vi "OnImageFrameAvailable Event Callback - TLCamera Main Color.vi"(4 "User Parameter":T3, 5 "Event Data":T4, 6 "Control Ref":refnum<k24>, 7 "Event Common Data":T5) -> ()   [LabVIEW 2015]
uses:
  C:/code/Host/Installer/Scientific Camera Interfaces/LabVIEW/32_bit/Library_X86/Thorlabs.TSI.TLCameraInterfaces.dll
  32_bit/Library_X86/Thorlabs.TSI.TLCameraInterfaces.dll
  SubVIs/Parameters Get & Set/Get Parameters/Get ColorFilterArrayPhase.vi
  C:/code/Host/Installer/Scientific Camera Interfaces/LabVIEW/32_bit/Library_X86/Thorlabs.TSI.ImageDataInterfaces.dll
  32_bit/Library_X86/Thorlabs.TSI.ImageDataInterfaces.dll
  SubVIs/Parameters Get & Set/Get Parameters/Get CameraSensorType.vi
  Controls/Color Modes.ctl
  C:/code/Host/Installer/Scientific Camera Interfaces/LabVIEW/32_bit/Library_X86/Thorlabs.TSI.Demosaicker.dll
  32_bit/Library_X86/Thorlabs.TSI.Demosaicker.dll
  C:/code/Host/Installer/Scientific Camera Interfaces/LabVIEW/32_bit/Library_X86/Thorlabs.TSI.ColorProcessor.dll
  32_bit/Library_X86/Thorlabs.TSI.ColorProcessor.dll
  C:/code/Host/Installer/Scientific Camera Interfaces/LabVIEW/32_bit/Library_X86/Thorlabs.TSI.ColorInterfaces.dll
  32_bit/Library_X86/Thorlabs.TSI.ColorInterfaces.dll
  SubVIs/Color/Color Processor References.ctl
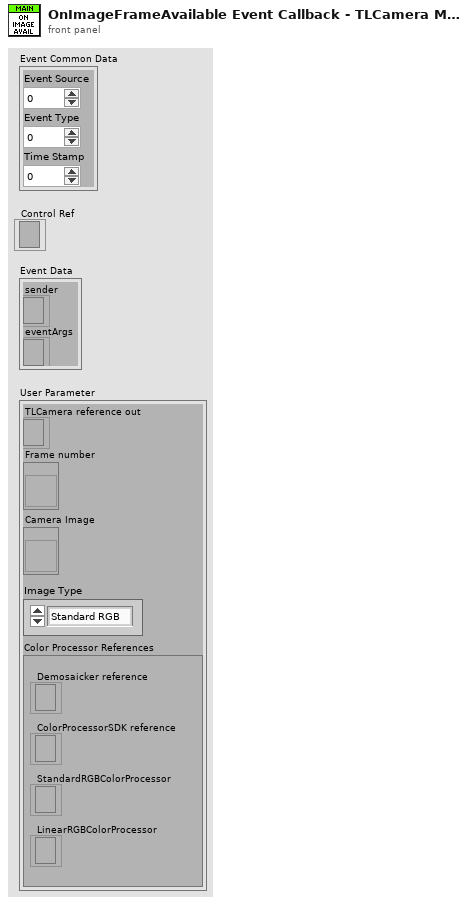
[diagram p1: front panel]
types:
  T1 = typedef "Color Modes.ctl" = enum16{"Standard RGB", "Linear RGB", "Unprocessed"}
  T2 = typedef "Color Processor References.ctl" = cluster{"Demosaicker reference":refnum<k24>, "ColorProcessorSDK reference":refnum<k24>, "StandardRGBColorProcessor":refnum<k24>, "LinearRGBColorProcessor":refnum<k24>}
  T3 = cluster{"TLCamera reference out":refnum<k24>, "Frame number":refnum<vi>, "Camera Image":refnum<vi>, "Image Type":T1, "Color Processor References":T2}
  T4 = cluster{"sender":refnum<k24>, "eventArgs":refnum<k24>}
  T5 = cluster{"Event Source":i32, "Event Type":u32, "Time Stamp":u32}
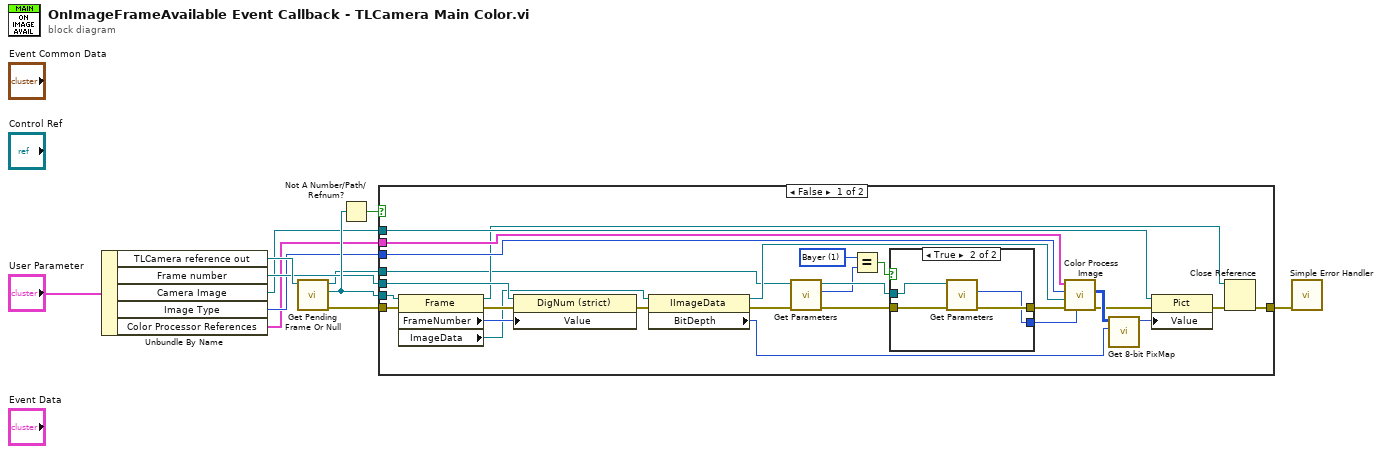
[diagram p0: block diagram]
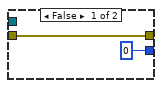
[diagram p2: hidden frame]
diagram:
  n1 = Unbundle By Name("User Parameter") -> ("TLCamera reference out"=w10:refnum<k24>, "Frame number"=w6:refnum<vi>, "Camera Image"=w2:refnum<vi>, "Image Type"=w5:T1, "Color Processor References"=w4:T2)
  n2 = call "Get Pending Frame Or Null.vi"("Thorlabs.TSI.TLCameraInterfaces.ITLCamera"=w10) -> ("error out"=w7:errorcluster, "Thorlabs.TSI.TLCameraInterfaces.Frame"=w8:refnum<k24>, "Thorlabs.TSI.TLCameraInterfaces.ITLCamera"=w3:refnum<k24>)  [unwired: 8 in]
  n3 = Not A Number/Path/Refnum?(number/path/refnum=w8) -> (NaN/Path/Refnum?=w9:bool)
  n4 = case shown="False" w9 {
    tunnel: w8 -> [w38 _]
    tunnel: w7 -> [w37 w45]
    tunnel: w6 -> [w36 _]
    tunnel: w5 -> [w33 _]
    tunnel: w4 -> [w32 _]
    tunnel: w3 -> [w18 _]
    tunnel: w2 -> [w23 _]
    tunnel: [w19 w45] -> w1
    frame False {
      w13 = 1 items=["Monochrome", "Bayer"] ("CameraSensorType")
      n5 = property class="Frame"(reference=w38, error in=w37) -> (reference out=w20:refnum<k24>, error out=w35:errorcluster, "FrameNumber"=w34:u32, "ImageData"=w29:refnum<k24>)
      n6 = property class="DigNum (strict)"(reference=w36, error in=w35, "Value"=w34) -> (error out=w27:errorcluster)  [unwired: 1 out]
      n7 = property class="IImageData"(reference=w29, error in=w27) -> (reference out=w28:refnum<k24>, error out=w17:errorcluster, "BitDepth"=w26:i32)
      n8 = call-poly "Get Parameters.vi"("error in (no error)"=w17, "Thorlabs.TSI.TLCameraInterfaces.ITLCamera"=w18) -> ("error out"=w15:errorcluster, "CameraSensorType"=w14:i32, "Thorlabs.TSI.TLCameraInterfaces.ITLCamera"=w16:refnum<k24>)  [unwired: 7 in]
      n9 = Equal?(x=w13, y=w14) -> (x = y?=w12:bool)
      n10 = case shown="True" w12 {
        tunnel: [w39 w44] -> w31
        tunnel: [0 ("ColorFilterArrayPhase") w43] -> w30
        tunnel: w16 -> [_ w42]
        tunnel: w15 -> [w39 w41]
        frame False {
        }
        frame True {
          n11 = call-poly "Get Parameters.vi"("error in (no error)"=w41, "Thorlabs.TSI.TLCameraInterfaces.ITLCamera"=w42) -> ("error out"=w44:errorcluster, "ColorFilterArrayPhase"=w43:i32)  [unwired: 7 in, 1 out]
        }
      }
      n12 = call "Color Process Image.vi"("Color Filter Array Phase"=w30, "error in (no error)"=w31, "Thorlabs.TSI.ImageDataInterfaces.IImageData"=w28, "Image Type"=w33, "Color Processor References"=w32) -> ("error out"=w24:errorcluster, "Color Data"=w25:u16[][][])  [unwired: 5 in]
      n13 = call "Get 8-bit PixMap.vi"("Original Bit depth"=w26, "Color Data"=w25) -> ("new picture"=w22:picture)  [unwired: 9 in]
      n14 = property class="Pict"(reference=w23, error in=w24, "Value"=w22) -> (error out=w21:errorcluster)  [unwired: 1 out]
      n15 = Close Reference(reference=w20, error in (no error)=w21) -> (error out=w19:errorcluster)
    }
    frame True {
    }
  }
  n16 = call <vilib>:"Simple Error Handler.vi"("error in (no error)"=w1) -> ()  [unwired: 4 in, 5 out]
